vi "Pneumatics_Begin.vi"   [LabVIEW 2014]
uses:
  <vilib>/Rock Robotics/WPI/Solenoid/WPI_SolenoidChannel.ctl
  <vilib>/Rock Robotics/WPI/Solenoid/WPI_SolenoidOpenSingle.vi
  <vilib>/Rock Robotics/WPI/Compressor/WPI_CompressorGetSetRefNum.vi
types:
  T1 = typedef "WPI_SolenoidChannel.ctl" = enum8{"Solenoid 0", "Solenoid 1", "Solenoid 2", "Solenoid 3", "Solenoid 4", "Solenoid 5", "Solenoid 6", "Solenoid 7", "Invalid"}
  T2 = typedef "WPI_CompressorDevRef.ctl" = cluster{"DevStatus":errorcluster, "Pneumatics Control Module":u8}
  T3 = typedef "WPI_SolenoidDevRef.ctl" = cluster{"DevStatus":errorcluster, "Pneumatics Control Module":u8, "Forward Solenoid Channel":T1, "Reverse Solenoid Channel":T1}
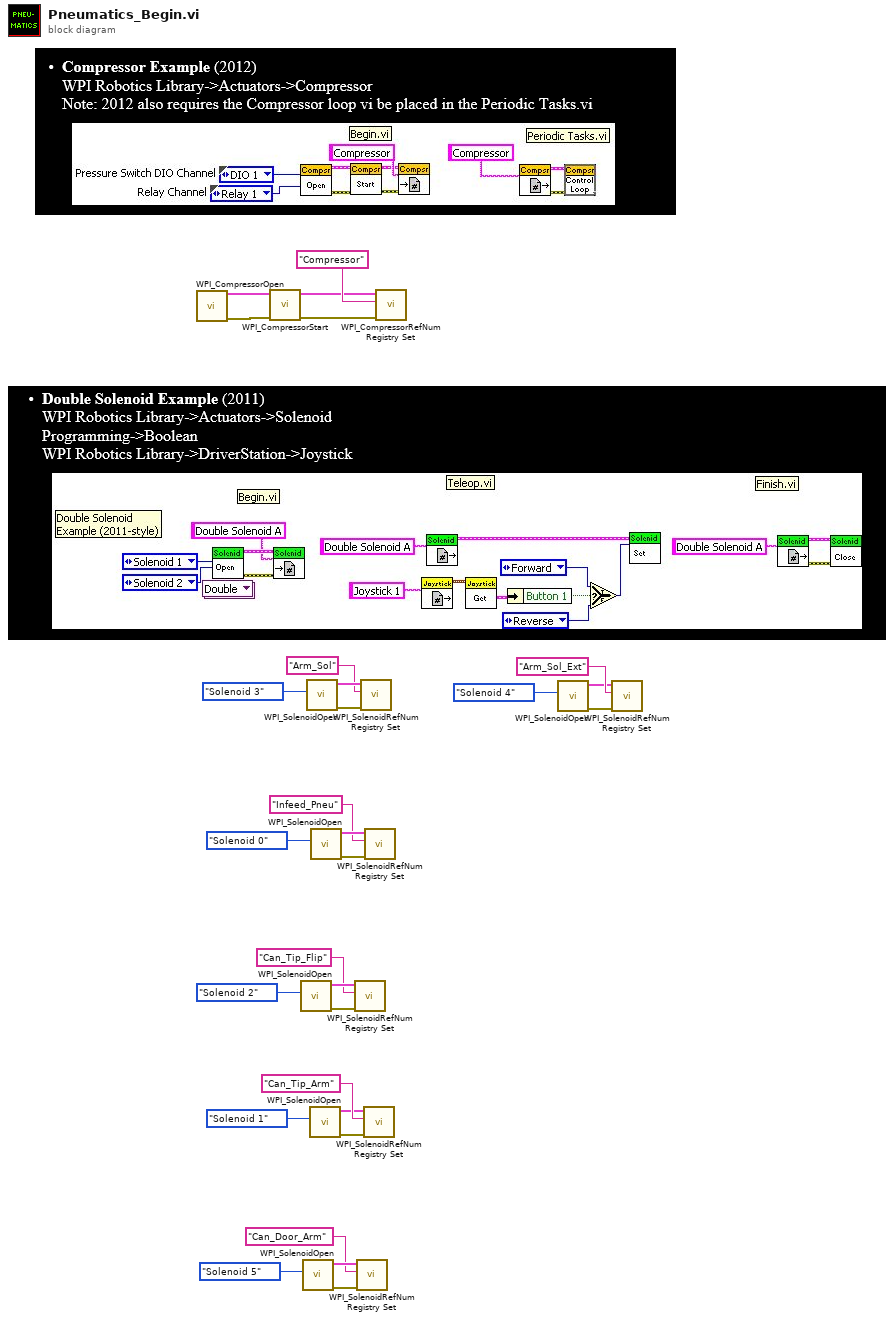
[diagram p0: block diagram]
diagram:
  n1 = call <vilib>:"WPI_CompressorOpen.vi"() -> ("CompressorDevRef"=w25:T2, "error out"=w28:errorcluster)  [unwired: 14 in]
  n2 = call <vilib>:"WPI_CompressorStart.vi"("error in (no error)"=w28, "CompressorDevRef"=w25) -> ("error out"=w29:errorcluster, "CompressorDevRef"=w26:T2)  [unwired: 8 in]
  n3 = call-poly <vilib>:"WPI_SolenoidOpen.vi"("Solenoid Channel"=WPI_SolenoidChannel."Solenoid 2" ("Forward Solenoid Channel")) -> ("error out"=w19:errorcluster, "SolenoidDevRef"=w20:T3)  [unwired: 9 in]
  n4 = call-poly <vilib>:"WPI_SolenoidOpen.vi"("Solenoid Channel"=WPI_SolenoidChannel."Solenoid 5" ("Forward Solenoid Channel")) -> ("error out"=w7:errorcluster, "SolenoidDevRef"=w8:T3)  [unwired: 9 in]
  n5 = call-poly <vilib>:"WPI_SolenoidOpen.vi"("Solenoid Channel"=WPI_SolenoidChannel."Solenoid 3" ("Forward Solenoid Channel")) -> ("error out"=w23:errorcluster, "SolenoidDevRef"=w24:T3)  [unwired: 9 in]
  n6 = call-poly <vilib>:"WPI_SolenoidOpen.vi"("Solenoid Channel"=WPI_SolenoidChannel."Solenoid 1" ("Forward Solenoid Channel")) -> ("error out"=w10:errorcluster, "SolenoidDevRef"=w9:T3)  [unwired: 9 in]
  n7 = call-poly <vilib>:"WPI_SolenoidOpen.vi"("Solenoid Channel"=WPI_SolenoidChannel."Solenoid 0" ("Forward Solenoid Channel")) -> ("error out"=w21:errorcluster, "SolenoidDevRef"=w22:T3)  [unwired: 9 in]
  n8 = call <vilib>:"WPI_SolenoidRefNum Registry Set.vi"("error in (no error)"=w19, "refnum name"="Can_Tip_Flip", "SolenoidDevRef"=w20) -> ()  [unwired: 7 in, 2 out]
  n9 = call <vilib>:"WPI_SolenoidRefNum Registry Set.vi"("error in (no error)"=w7, "refnum name"="Can_Door_Arm", "SolenoidDevRef"=w8) -> ()  [unwired: 7 in, 2 out]
  n10 = call <vilib>:"WPI_SolenoidRefNum Registry Set.vi"("error in (no error)"=w23, "refnum name"="Arm_Sol", "SolenoidDevRef"=w24) -> ()  [unwired: 7 in, 2 out]
  n11 = call <vilib>:"WPI_SolenoidRefNum Registry Set.vi"("error in (no error)"=w10, "refnum name"="Can_Tip_Arm", "SolenoidDevRef"=w9) -> ()  [unwired: 7 in, 2 out]
  n12 = call <vilib>:"WPI_SolenoidRefNum Registry Set.vi"("error in (no error)"=w21, "refnum name"="Infeed_Pneu", "SolenoidDevRef"=w22) -> ()  [unwired: 7 in, 2 out]
  n13 = call <vilib>:"WPI_CompressorRefNum Registry Set.vi"("error in (no error)"=w29, "refnum name"="Compressor", "CompressorDevRef"=w26) -> ()  [unwired: 7 in, 2 out]
  n14 = call-poly <vilib>:"WPI_SolenoidOpen.vi"("Solenoid Channel"=WPI_SolenoidChannel."Solenoid 4" ("Forward Solenoid Channel")) -> ("error out"=w2:errorcluster, "SolenoidDevRef"=w1:T3)  [unwired: 9 in]
  n15 = call <vilib>:"WPI_SolenoidRefNum Registry Set.vi"("error in (no error)"=w2, "refnum name"="Arm_Sol_Ext", "SolenoidDevRef"=w1) -> ()  [unwired: 7 in, 2 out]
